vi "GetButtonValue.vi"(8 "error in (no error)":errorcluster, 10 "label":string, 11 "Buttons":refnum<vi>[](array[refnum])) -> (0 "error out":errorcluster, 2 "Value":bool, 3 "Buttons out":refnum<vi>[](array[refnum]))   [LabVIEW 2018, in "CarWashTestCases.lvclass"]
uses:
  CarWashTestCases.lvclass
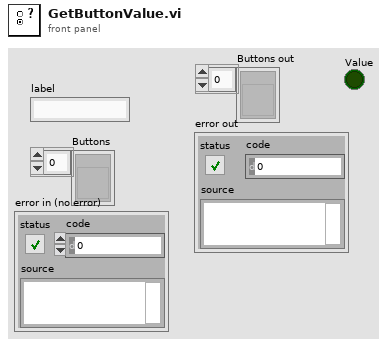
[diagram p1: front panel]
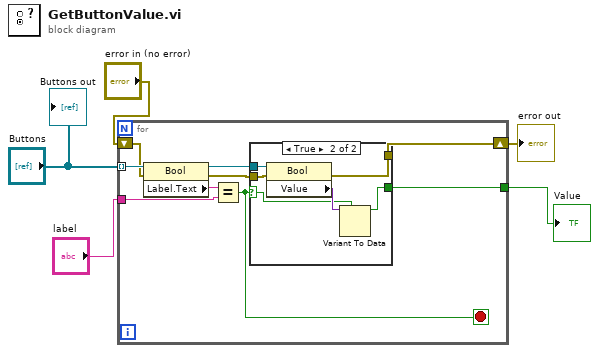
[diagram p0: block diagram]
diagram:
  n1 = for {
    tunnel: "Buttons" -> [w11] mode=indexing
    tunnel: "label" -> [w13]
    shift-right: [w8] -> w2
    shift-left: "error in (no error)" -> [w10]
    tunnel: [w7] -> w1
    stop <- w6 stop-if-true
    n2 = property class="Bool"(reference=w11, error in=w10) -> (reference out=w12:refnum<vi>, error out=w9:errorcluster, "Label.Text"=w14:string)
    n3 = Equal?(x=w14, y=w13) -> (x = y?=w6:bool)
    n4 = case shown="True" w6 {
      selector: w6 -> [_ w17]
      tunnel: w12 -> [_ w21]
      tunnel: w9 -> [w15 w20]
      tunnel: [w15 w19] -> w8
      tunnel: [_ w16] -> w7
      frame False {
      }
      frame True {
        n5 = property class="Bool"(reference=w21, error in=w20) -> (error out=w19:errorcluster, "Value"=w18:variant)  [unwired: 1 out]
        n6 = Variant To Data(type=w17, Variant=w18) -> (data=w16:bool)  [unwired: 1 in, 1 out]
      }
    }
  }
  "error out" <- w2
  "Value" <- w1
  "Buttons out" <- "Buttons"
